vi "visualize_wire.vi"(10 "small angle":sgl, 11 "large axis angle":sgl) -> (3 "3D Picture 3":refnum<vi>(3d-picture))   [LabVIEW 2016]
uses:
  <vilib>/picture/3D Picture Control/Object/Create Object (name).vi
  <vilib>/picture/3D Picture Control/NI_3D Picture Control.lvlib
panel:
  in  "y":i32
  out "error out":errorcluster
  in  "error in (no error)":errorcluster
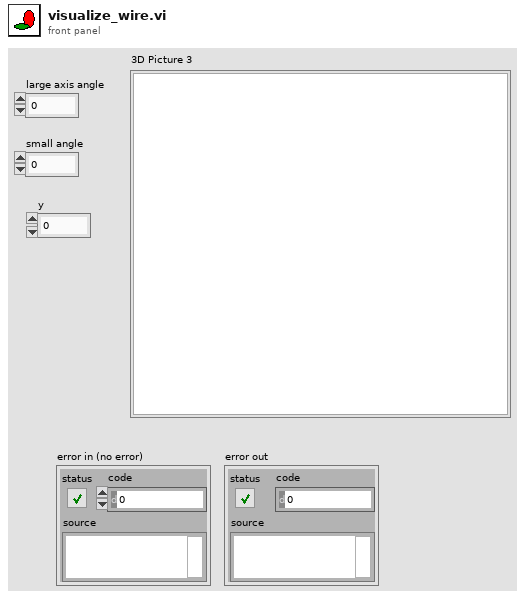
[diagram p1: front panel]
types:
  T1 = cluster{"Red":sgl, "Green":sgl, "Blue":sgl, "Alpha":sgl}
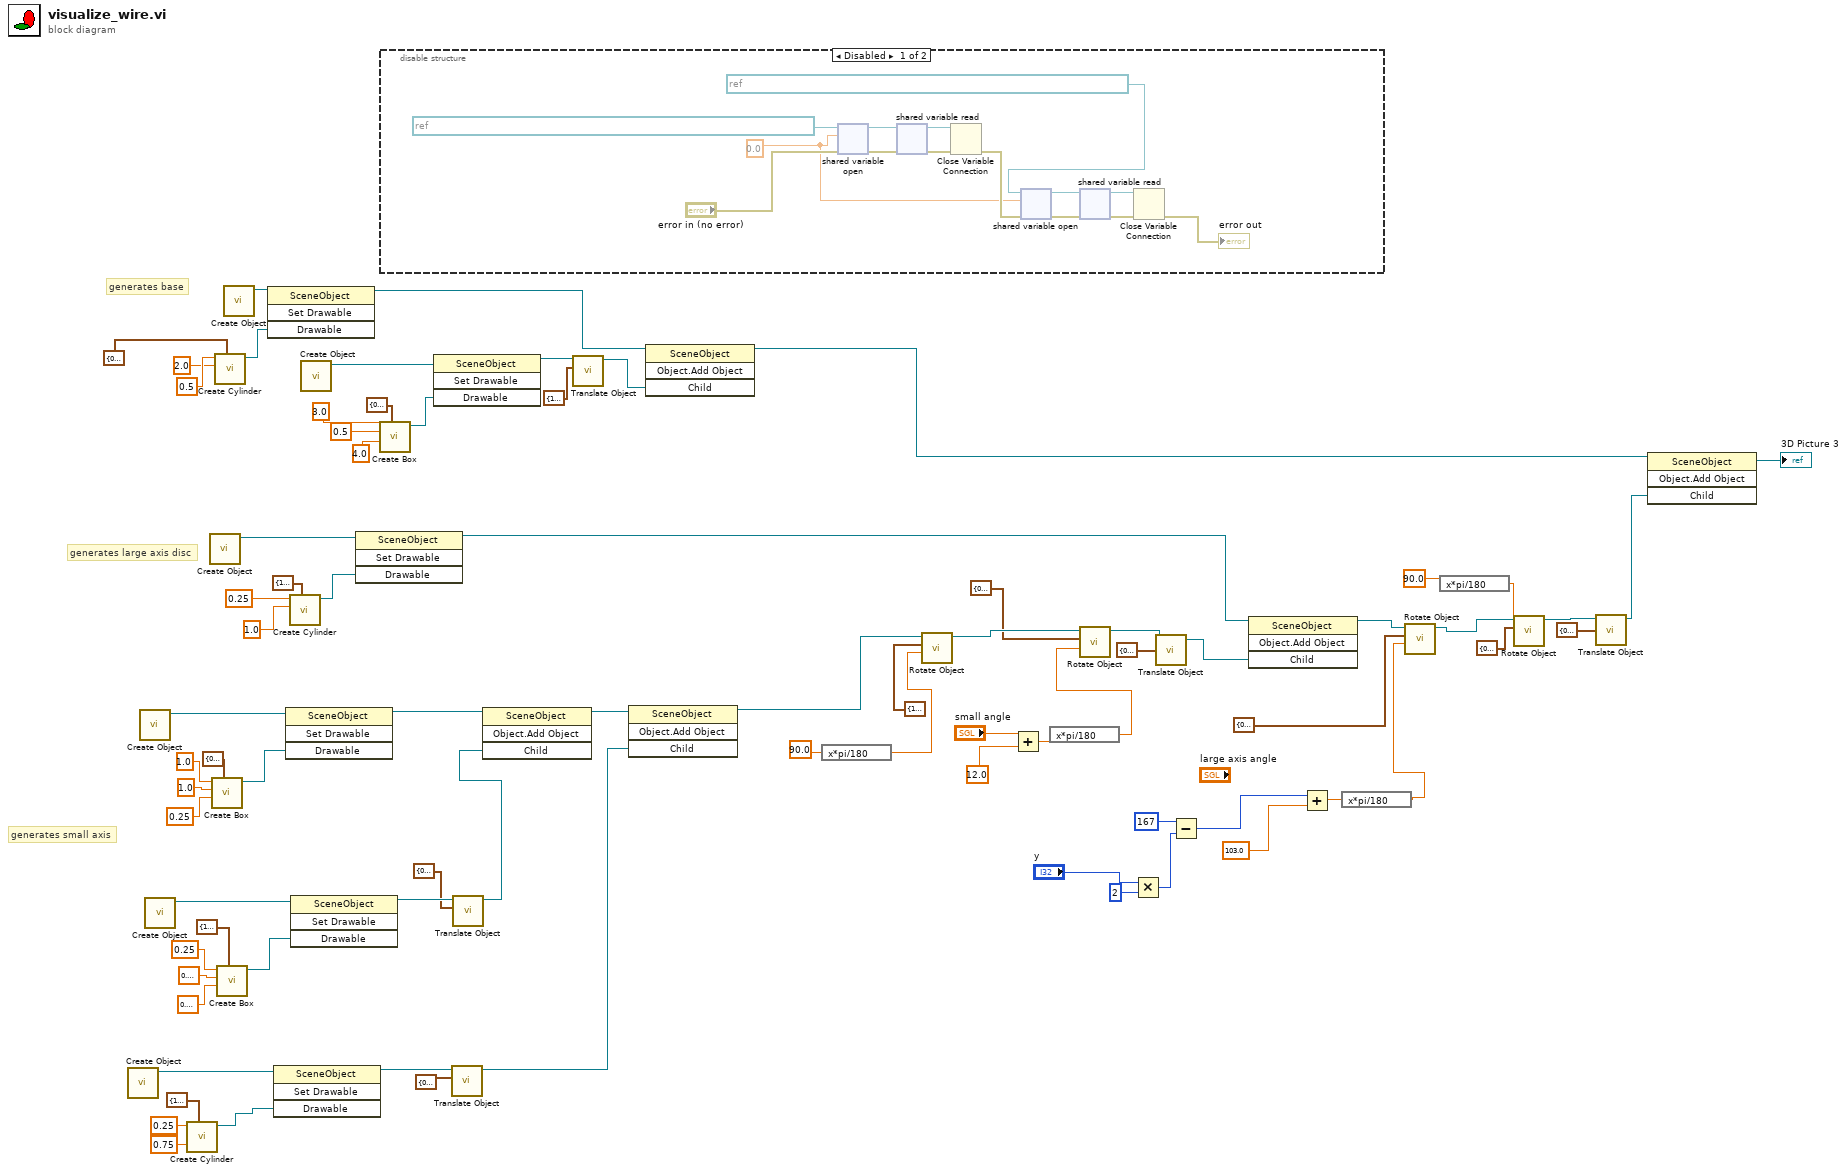
[diagram p0: block diagram]
diagram:
  # "generates small axis"
  # "generates large axis disc"
  # "generates base"
  n1 = call-poly <vilib>:"Create Object.vi"() -> ("Scene:New Object"=w65:refnum<vi>)  [unwired: 10 in, 1 out]
  n2 = call-poly <vilib>:"Create Object.vi"() -> ("Scene:New Object"=w78:refnum<vi>)  [unwired: 10 in, 1 out]
  n3 = call-poly <vilib>:"Create Object.vi"() -> ("Scene:New Object"=w67:refnum<vi>)  [unwired: 10 in, 1 out]
  n4 = call <vilib>:"Create Cylinder.vi"("Color"=T1 {"Red"=1.0, "Green"=1.0, "Blue"=1.0, "Alpha"=1.0}, "Radius"=sgl 0.75, "Height"=sgl 0.25) -> ("New Cylinder Refnum"=w64:refnum<vi>)  [unwired: 7 in, 1 out]
  n5 = call-poly <vilib>:"Create Object.vi"() -> ("Scene:New Object"=w50:refnum<vi>)  [unwired: 10 in, 1 out]
  n6 = call <vilib>:"Create Box.vi"("Color"=T1 {"Red"=0.0, "Green"=1.0, "Blue"=0.0, "Alpha"=1.0}, "Length Z"=sgl 0.25, "Length Y"=sgl 1.0, "Length X"=sgl 1.0) -> ("New Box Refnum"=w74:refnum<vi>)  [unwired: 6 in, 1 out]
  n7 = call <vilib>:"Create Cylinder.vi"("Color"=T1 {"Red"=0.8, "Green"=0.5, "Blue"=0.2, "Alpha"=1.0}, "Radius"=sgl 2.0, "Height"=sgl 0.5) -> ("New Cylinder Refnum"=w35:refnum<vi>)  [unwired: 7 in, 1 out]
  n8 = call <vilib>:"Create Box.vi"("Color"=T1 {"Red"=1.0, "Green"=1.0, "Blue"=0.0, "Alpha"=1.0}, "Length Z"=sgl 0.1, "Length Y"=sgl 0.1, "Length X"=sgl 0.25) -> ("New Box Refnum"=w71:refnum<vi>)  [unwired: 6 in, 1 out]
  n9 = call-poly <vilib>:"Create Object.vi"() -> ("Scene:New Object"=w34:refnum<vi>)  [unwired: 10 in, 1 out]
  n10 = invoke class="SceneObject" method="Set Drawable"(reference=w34, "Drawable"=w35) -> (reference out=w24:refnum<vi>)  [unwired: 2 in, 3 out]
  n11 = invoke class="SceneObject" method="Set Drawable"(reference=w65, "Drawable"=w64) -> (reference out=w59:refnum<vi>)  [unwired: 2 in, 3 out]
  n12 = invoke class="SceneObject" method="Set Drawable"(reference=w78, "Drawable"=w74) -> (reference out=w66:refnum<vi>)  [unwired: 2 in, 3 out]
  n13 = call <vilib>:"Create Cylinder.vi"("Color"=T1 {"Red"=1.0, "Green"=1.0, "Blue"=1.0, "Alpha"=1.0}, "Radius"=sgl 1.0, "Height"=sgl 0.25 ("Length Z")) -> ("New Cylinder Refnum"=w48:refnum<vi>)  [unwired: 7 in, 1 out]
  n14 = invoke class="SceneObject" method="Set Drawable"(reference=w67, "Drawable"=w71) -> (reference out=w56:refnum<vi>)  [unwired: 2 in, 3 out]
  n15 = call-poly <vilib>:"Create Object.vi"() -> ("Scene:New Object"=w33:refnum<vi>)  [unwired: 10 in, 1 out]
  n16 = invoke class="SceneObject" method="Set Drawable"(reference=w50, "Drawable"=w48) -> (reference out=w45:refnum<vi>)  [unwired: 2 in, 3 out]
  n17 = call <vilib>:"Create Box.vi"("Color"=T1 {"Red"=0.8, "Green"=0.5, "Blue"=0.2, "Alpha"=1.0}, "Length Z"=sgl 4.0, "Length Y"=sgl 3.0, "Length X"=sgl 0.5) -> ("New Box Refnum"=w30:refnum<vi>)  [unwired: 6 in, 1 out]
  n18 = disable-structure shown="Disabled" {
    frame Disabled {
      w82 = sgl 0.0 ("Angle")
      n19 = shared-variable-open(refnum<k21> "ni.var.psp://housesoftheholy/Attocube 3DR/axis 1%3A current position" ("shared variable refnum in"), "error in (no error)", w82) -> (w92:refnum<k21>, w91:errorcluster)  [unwired: 1 in]
      n20 = shared-variable-read(w92, w91) -> (w81:refnum<k21>, w90:errorcluster)  [unwired: 2 out]
      n21 = Close Variable Connection(8:w90, 11:w81) -> (0:w85:errorcluster)
      n22 = shared-variable-open(refnum<k21> "ni.var.psp://housesoftheholy/Attocube 3DR/axis 2%3A current position" ("shared variable refnum in"), w85, w82) -> (w86:refnum<k21>, w87:errorcluster)  [unwired: 1 in]
      n23 = shared-variable-read(w86, w87) -> (w80:refnum<k21>, w88:errorcluster)  [unwired: 2 out]
      n24 = Close Variable Connection(8:w88, 11:w80) -> (0:→"error out":errorcluster)
    }
    frame Enabled {
    }
  }
  n25 = invoke class="SceneObject" method="Set Drawable"(reference=w33, "Drawable"=w30) -> (reference out=w26:refnum<vi>)  [unwired: 2 in, 3 out]
  n26 = call <vilib>:"Translate Object.vi"("Translation"=cluster{"X":sgl, "Y":sgl, "Z":sgl} {"X"=0.0, "Y"=0.0, "Z"=-0.25}, "Scene.Object In"=w59) -> ("Scene.Object Out"=w57:refnum<vi>)  [unwired: 8 in, 1 out]
  n27 = call <vilib>:"Translate Object.vi"("Translation"=cluster{"X":sgl, "Y":sgl, "Z":sgl} {"X"=0.4, "Y"=0.0, "Z"=0.1}, "Scene.Object In"=w56) -> ("Scene.Object Out"=w54:refnum<vi>)  [unwired: 8 in, 1 out]
  n28 = invoke class="SceneObject" method="Object.Add Object"(reference=w66, "Child"=w54) -> (reference out=w60:refnum<vi>)  [unwired: 2 in, 3 out]
  n29 = call <vilib>:"Translate Object.vi"("Translation"=cluster{"X":sgl, "Y":sgl, "Z":sgl} {"X"=1.0, "Y"=0.0, "Z"=2.0}, "Scene.Object In"=w26) -> ("Scene.Object Out"=w25:refnum<vi>)  [unwired: 8 in, 1 out]
  n30 = invoke class="SceneObject" method="Object.Add Object"(reference=w60, "Child"=w57) -> (reference out=w40:refnum<vi>)  [unwired: 2 in, 3 out]
  n31 = invoke class="SceneObject" method="Object.Add Object"(reference=w24, "Child"=w25) -> (reference out=w22:refnum<vi>)  [unwired: 2 in, 3 out]
  n32 = expression code="x*pi/180"(sgl 90.0 ("small axis angle")) -> (w51:sgl)
  n33 = call <vilib>:"Rotate Object.vi"("Angle"=w51, "Axis"=cluster{"X":sgl, "Y":sgl, "Z":sgl} {"X"=1.0, "Y"=0.0, "Z"=0.0} ("rotate small axis"), "Scene.Object In"=w40) -> ("Scene.Object Out"=w42:refnum<vi>)  [unwired: 7 in, 1 out]
  n34 = Add(x="small angle", y=sgl 12.0 ("y 2")) -> (x+y=w10:sgl)
  n35 = expression code="x*pi/180"(w10) -> (w9:sgl)
  n36 = call <vilib>:"Rotate Object.vi"("Angle"=w9, "Axis"=cluster{"X":sgl, "Y":sgl, "Z":sgl} {"X"=0.0, "Y"=1.0, "Z"=0.0} ("small axis"), "Scene.Object In"=w42) -> ("Scene.Object Out"=w39:refnum<vi>)  [unwired: 7 in, 1 out]
  n37 = Multiply(x="y", y=2) -> (x*y=w2:i32)
  n38 = call <vilib>:"Translate Object.vi"("Translation"=cluster{"X":sgl, "Y":sgl, "Z":sgl} {"X"=0.0, "Y"=0.5, "Z"=-1.0} ("translate small axis"), "Scene.Object In"=w39) -> ("Scene.Object Out"=w37:refnum<vi>)  [unwired: 8 in, 1 out]
  n39 = Subtract(x=167, y=w2) -> (x-y=w1:i32)
  n40 = invoke class="SceneObject" method="Object.Add Object"(reference=w45, "Child"=w37) -> (reference out=w44:refnum<vi>)  [unwired: 2 in, 3 out]
  n41 = Add(x=w1, y=sgl 103.0) -> (x+y=w8:sgl)
  n42 = expression code="x*pi/180"(w8) -> (w7:sgl)
  n43 = call <vilib>:"Rotate Object.vi"("Angle"=w7, "Axis"=cluster{"X":sgl, "Y":sgl, "Z":sgl} {"X"=0.0, "Y"=0.0, "Z"=1.0} ("Large axis"), "Scene.Object In"=w44) -> ("Scene.Object Out"=w20:refnum<vi>)  [unwired: 7 in, 1 out]
  n44 = expression code="x*pi/180"(sgl 90.0 ("Angle")) -> (w14:sgl)
  n45 = call <vilib>:"Rotate Object.vi"("Angle"=w14, "Axis"=cluster{"X":sgl, "Y":sgl, "Z":sgl} {"X"=0.0, "Y"=1.0, "Z"=0.0}, "Scene.Object In"=w20) -> ("Scene.Object Out"=w19:refnum<vi>)  [unwired: 7 in, 1 out]
  n46 = call <vilib>:"Translate Object.vi"("Translation"=cluster{"X":sgl, "Y":sgl, "Z":sgl} {"X"=0.5, "Y"=0.0, "Z"=3.0}, "Scene.Object In"=w19) -> ("Scene.Object Out"=w18:refnum<vi>)  [unwired: 8 in, 1 out]
  n47 = invoke class="SceneObject" method="Object.Add Object"(reference=w22, "Child"=w18) -> (reference out=→"3D Picture 3":refnum<vi>)  [unwired: 2 in, 3 out]
